vi "Stop Splash.vi"(8 "error in (no error)":errorcluster, 11 "Splash Screen ViewManager in":refnum<class "Splash Screen ViewManager.lvclass">) -> (0 "error out":errorcluster, 3 "Splash Screen ViewManager out":refnum<class "Splash Screen ViewManager.lvclass">)   [LabVIEW 2019, in "Splash Screen ViewManager.lvclass"]
uses:
  <vilib>/gpm_packages/@cs/Car-wash/Source/Splash Screen ViewManager/Splash Screen ViewManager.lvclass
  C:/Program Files/National Instruments/LabVIEW 2019/vi.lib/gpm_packages/@cs/mva-viewable/Source/IViewManager/IViewManager/IViewManager.lvclass
  <vilib>/gpm_packages/@cs/mva-viewable/Source/IViewManager/IViewManager/IViewManager.lvclass/IViewManager.ctl
  <vilib>/gpm_packages/@cs/Car-wash/Source/Splash Screen ViewManager/Splash Screen ViewManager.lvclass/Splash Screen ViewManager.ctl
  <vilib>/gpm_packages/@cs/mva-viewable/Source/IViewable/IViewable Messages/Insert Front Panel Msg/Insert Front Panel Msg.lvclass/Insert Front Panel Msg.ctl
  <vilib>/ActorFramework/Message Enqueuer/Message Enqueuer.lvclass/Message Enqueuer.ctl
  <vilib>/ActorFramework/Message Enqueuer/Enqueue.vi
  <vilib>/gpm_packages/@cs/mva-viewable/Source/IViewable/IViewable Messages/Insert Front Panel Msg/Insert Front Panel Msg.lvclass
  C:/Program Files/National Instruments/LabVIEW 2019/vi.lib/ActorFramework/Message/Message.lvclass
  <vilib>/ActorFramework/Message Priority Queue/Priority Enqueue.vi
  <vilib>/gpm_packages/@cs/mva-viewable/Source/IViewManager/IViewManager/IViewManager.lvclass
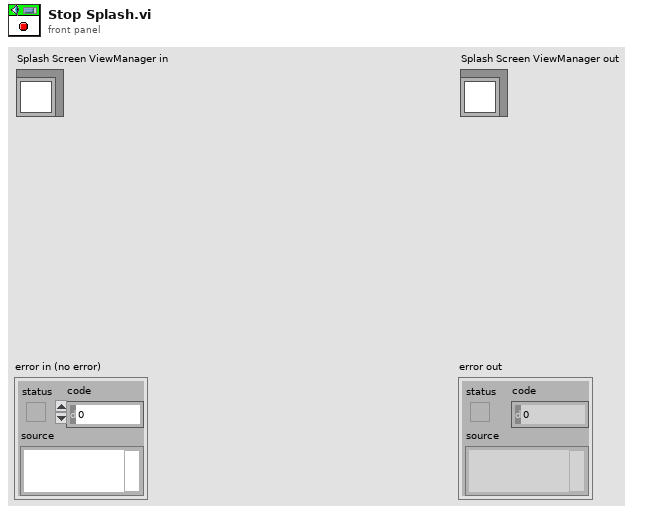
[diagram p1: front panel]
types:
  T1 = typedef "IViewable.lvlib/ProtectedSubpanel.lvclass/Protected Subpanel Reference.ctl" = refnum<data-value>
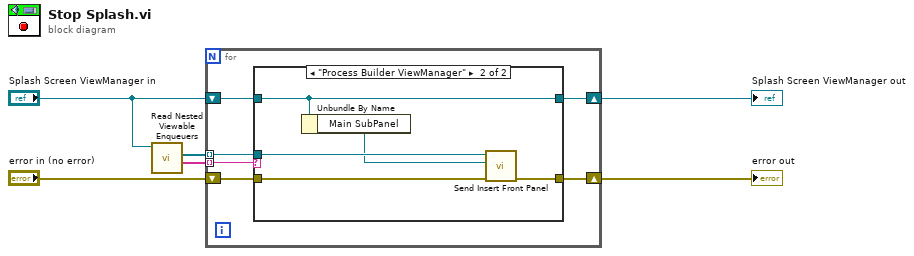
[diagram p0: block diagram]
diagram:
  n1 = call <vilib>:"Read Nested Viewable Enqueuers.vi"("IViewManager in"="Splash Screen ViewManager in") -> ("Viewable Names"=w5:string[], "Nested Viewable Enqueuers"=w6:refnum<class "Message Enqueuer.lvclass">[])  [unwired: 9 in]
  n2 = for {
    tunnel: w6 -> [w10] mode=indexing
    tunnel: w5 -> [w7] mode=indexing
    shift-right: [w8] -> w3
    shift-left: "Splash Screen ViewManager in" -> [w9]
    shift-right: [w11] -> w1
    shift-left: "error in (no error)" -> [w12]
    n3 = case shown="\"Process Builder ViewManager\"" w7 {
      tunnel: w12 -> [w13 w19]
      tunnel: [w13 w18] -> w11
      tunnel: w10 -> [_ w17]
      tunnel: [w14 w16] -> w8
      tunnel: w9 -> [w14 w16]
      frame Default {
      }
      frame "Process Builder ViewManager" {
        n4 = Unbundle By Name(w16) -> ("Main SubPanel"=w15:T1)
        n5 = call <vilib>:"Send Insert Front Panel.vi"("error in (no error)"=w19, "Protected Subpanel"=w15, "Message Enqueuer"=w17) -> ("error out"=w18:errorcluster)  [unwired: 7 in, 1 out]
      }
    }
  }
  "error out" <- w1
  "Splash Screen ViewManager out" <- w3
